vi "Run Best Optimisation Parameters.vi"(8 "error in (no error)":errorcluster, 11 "Monkey in":refnum<class "Monkey.lvclass">) -> (0 "error out":errorcluster, 2 "Best Parameters":string[][](array[string]), 3 "Monkey out":refnum<class "Monkey.lvclass">)   [LabVIEW 2020, in "TALOS.lvlib" / "Monkey.lvlib" / "Monkey.lvclass"]
uses:
  Monkey.lvclass
  Monkey.lvclass/Monkey.ctl
  Ancestor/Ancestor/Ancestor.lvclass/Ancestor.ctl
  Support VIs/Generate Error.vi
  FGV/Error Memory/Get Error Description.vi
  Support VIs/Get PC name.vi
  Ancestor/Ancestor/Read ID.vi
  Support VIs/Get Class Name.vi
  <vilib>/Utility/error.llb/Clear Errors.vi
  FGV/Error Memory/Error Memory Core.vi
  <vilib>/AdvancedString/Delimited String to 1D String Array.vi
  Support VIs/Circus Root Path.vi
  FGV/Error Memory/Error Crt Lvl checker.vi
  FGV/Error Memory/Error Memory Core.vi/40c8088d-b597-4017-91af-faa98e00292e.vi
  FGV/Error Memory/Error Memory Core.vi/d4a3ab98-063c-4e44-b43d-fbdcfe6c2be2.vi
  Support VIs/Global Memory.vi
  <vilib>/Utility/LVClass/Get LV Class Name.vi
  Support VIs/Is in Packed Library.vi
  Support VIs/TALOS Root path.vi
  Support VIs/Read CSV worksheet.vi
  Support VIs/Global Constants.vi
  <vilib>/Utility/error.llb/General Error Handler.vi
  Support VIs/Error Log.vi
  Ancestor/Ancestor/Ancestor.lvclass
  <vilib>/Comparison/Equal/Equal Functor/Equal Functor.lvclass
  Run Utilities/Run Block/Run Block.lvclass
  Run Utilities/Optimiser Cell/Optimiser Cell.lvclass
  Run Utilities/Run Instance/Run Instance.lvclass
  Run Utilities/Cell/Schedule Cell.lvclass
  TALOS.lvlib
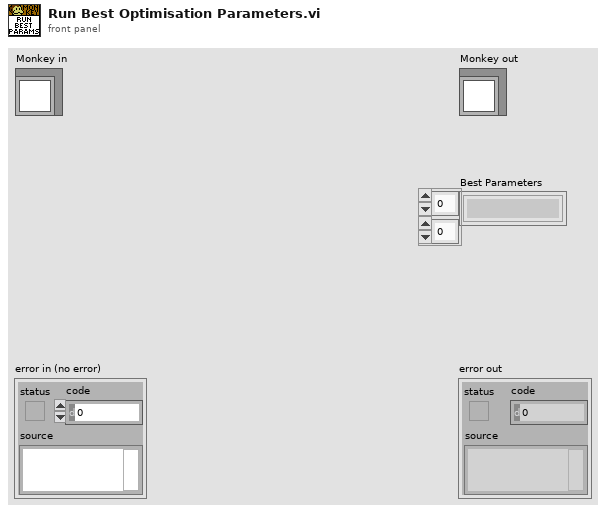
[diagram p1: front panel]
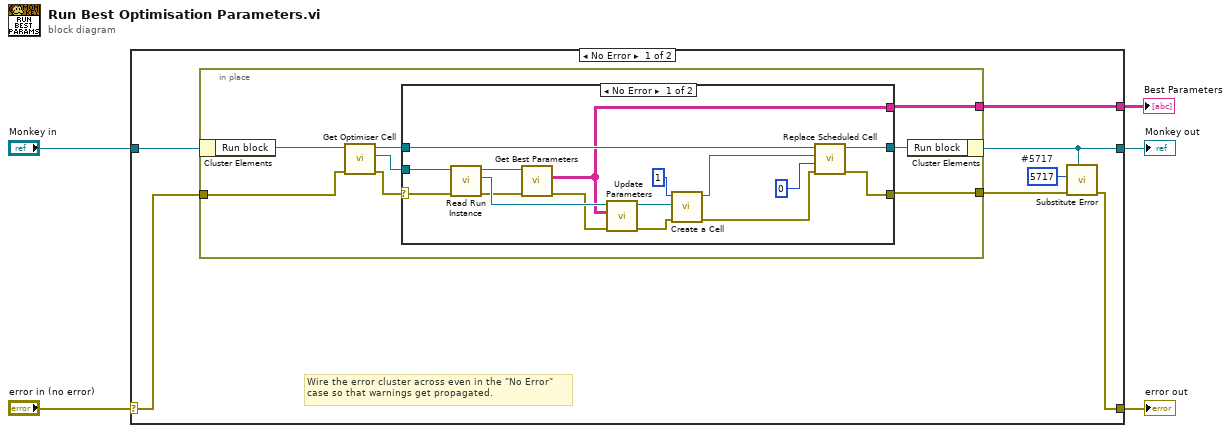
[diagram p0: block diagram]
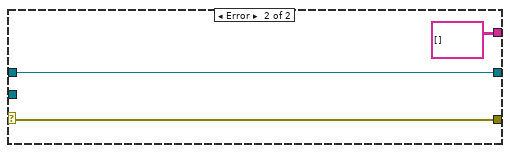
[diagram p2: hidden frame]
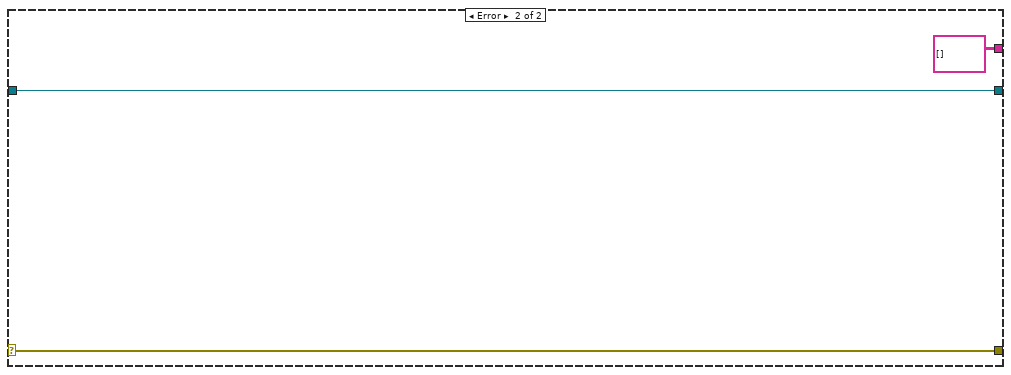
[diagram p3: hidden frame]
diagram:
  n1 = case shown="No Error" "error in (no error)" {
    selector: "error in (no error)" -> [w12 w42]
    tunnel: [w8 w42] -> w4
    tunnel: [w10 w41] -> w2
    tunnel: "Monkey in" -> [w11 w41]
    tunnel: [w6 string[][] [] ("Best Parameters")] -> w1
    frame No Error {
      w7 = 5717  # #5717
      # "Wire the error cluster across even in the \"No Error\"\ncase so that warnings get propagated."
      n2 = in-place {
        in-place-border: w12 -> [w20]
        in-place-border: [w14] -> w9
        in-place-border: [w13] -> w6
        n3 = in-place-cluster #1(w11) -> ("Run block"=w19:refnum<class "Run Block.lvclass">)
        n4 = call-dynamic "Get Optimiser Cell.vi"("error in (no error)"=w20, "Run Block in"=w19) -> ("error out"=w17:errorcluster, "Optimiser Cell"=w16:refnum<class "Optimiser Cell.lvclass">, "Run Block out"=w18:refnum<class "Run Block.lvclass">)  [unwired: 7 in]
        n5 = case shown="No Error" w17 {
          selector: w17 -> [w27 w38]
          tunnel: w18 -> [w36 w39]
          tunnel: w16 -> [w35 _]
          tunnel: [w28 w39] -> w15
          tunnel: [w26 w38] -> w14
          tunnel: [w22 string[][] [] ("Best Parameters")] -> w13
          frame No Error {
            n6 = call-dynamic "Read Run Instance.vi"("error in (no error)"=w27, "Schedule Cell in"=w35) -> ("error out"=w24:errorcluster, "Run Instance"=w25:refnum<class "Run Instance.lvclass">, "Schedule Cell out"=w23:refnum<class "Optimiser Cell.lvclass">)  [unwired: 7 in]
            n7 = call-dynamic "Get Best Parameters.vi"("error in (no error)"=w24, "Run Optimiser in"=w23) -> ("error out"=w21:errorcluster, "Best Parameters"=w22:string[][])  [unwired: 7 in, 1 out]
            n8 = call-dynamic "Update Parameters.vi"("error in (no error)"=w21, "Parameters"=w22, "Run Instance in"=w25) -> ("error out"=w32:errorcluster, "Run Instance out"=w33:refnum<class "Run Instance.lvclass">)  [unwired: 6 in, 1 out]
            n9 = call "Create a Cell.vi"("error in (no error)"=w32, "Run Instance"=w33, "Repetitions"=u32 1) -> ("error out"=w30:errorcluster, "Schedule Cell out"=w31:refnum<class "Schedule Cell.lvclass">)  [unwired: 7 in]
            n10 = call-dynamic "Replace Scheduled Cell.vi"("error in (no error)"=w30, "Index"=0, "Schedule Cell"=w31, "Run Block in"=w36) -> ("error out"=w26:errorcluster, "Run Block out"=w28:refnum<class "Run Block.lvclass">)  [unwired: 6 in]
          }
          frame Error {
          }
        }
        n11 = in-place-cluster #1("Run block"=w15) -> (w10:refnum<class "Monkey.lvclass">)
      }
      n12 = call "Substitute Error.vi"("LabVIEW Object"=w10, "error in (no error)"=w9, "Error Code"=w7) -> ("error out"=w8:errorcluster)  [unwired: 8 in]
    }
    frame Error {
    }
  }
  "error out" <- w4
  "Monkey out" <- w2
  "Best Parameters" <- w1
